vi "Boxplot.vi"(1 "Box Plot Ref":refnum<vi>, 2 "Data":dbl[][](array[numeric]), 3 "error in (no error)":errorcluster) -> (7 "Box Plot":cluster{dbl[], dbl[]}[](graph), 9 "error out":errorcluster)   [LabVIEW 2023]
doc: "Creates an Exploratory Data Analysis (EDA) boxplot of data. The boxplot consists of rectangles that represent the upper quartile, median, and lower quartile, whiskers that provide information about the distribution of the data, and 'X' symbols that indicate outliers."
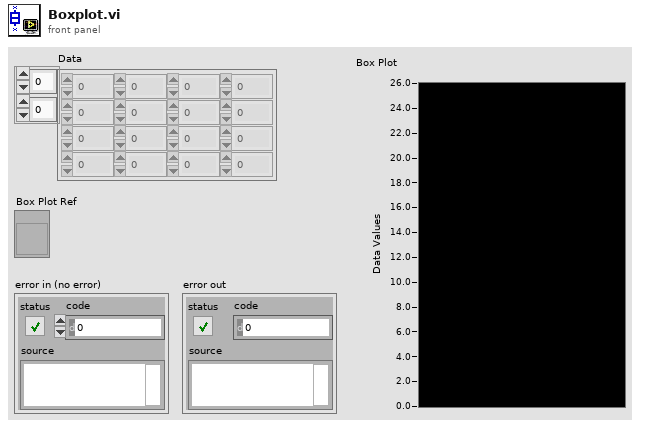
[diagram p1: front panel]
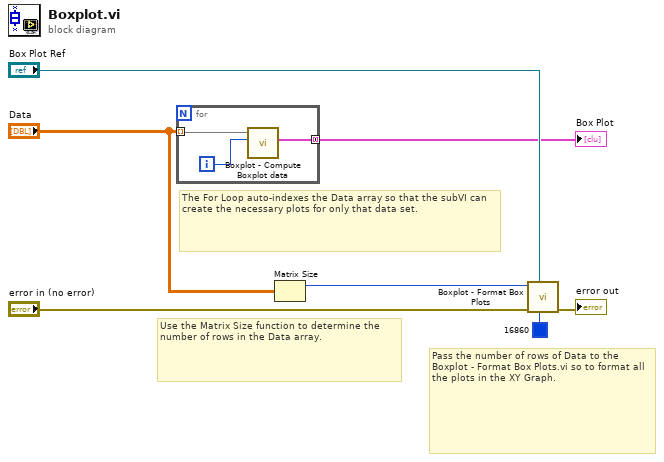
[diagram p0: block diagram]
diagram:
  # "Use the Matrix Size function to determine the number of rows in the Data array."
  # "Pass the number of rows of Data to the Boxplot - Format Box Plots.vi so to format all the plots in the XY Graph."
  # "The For Loop auto-indexes the Data array so that the subVI can create the necessary plots for only that data set."
  n1 = for {
    tunnel: "Data" -> [w9] mode=indexing
    tunnel: [w8] -> w3 mode=concatenating
    i -> [w10]
    n2 = call "Boxplot - Compute Boxplot data.vi"("Plot number"=w10, "Raw data"=w9) -> ("Boxplot"=w8:cluster{dbl[], dbl[]}[])  [unwired: 9 in]
  }
  "Box Plot" <- w3
  n3 = Matrix Size(0:"Data") -> (1:w1:i32)  [unwired: 1 out]
  n4 = call "Boxplot - Format Box Plots.vi"("Plot Color"=u32 16860 ("Plot.Plot Color"), "XY Graph"="Box Plot Ref", "error in (no error)"="error in (no error)", "Number of Plots"=w1) -> ("error out"=→"error out":errorcluster)  [unwired: 7 in]
